vi "Request Data.vi"(6 "Qualifier":string, 8 "error in":errorcluster, 9 "notifier":refnum<notifier>, 10 "Data to Send":string, 11 "PRM in":refnum<class "PRM.lvclass">) -> (0 "error out":errorcluster, 3 "PRM out":refnum<class "PRM.lvclass">)   [LabVIEW 2019, in "PRM.lvlib" / "PRM.lvclass"]
doc: "Data to Send is a required input that describes the measurement or query function to be performed\nQualifier is a secondary variable used in the event that specificity must be provided to the query function\n****Note****\nIf further specificity is required, the qualifier must be used in a comma delimited format to increase the overall variable count. Additional specificity must be provided by the child class and interpreted by the automated call.\n\nnotifier is a single variant notifier in which the instrument will send the data notification to the automated tool."
uses:
  Library/PRM.lvclass
  C:/Users/Public/Documents/Development/builds/Instruments/Instruments.lvlibp/Library/Instruments.lvclass
  C:/Users/Public/Documents/Development/builds/Engine/Monitored Actor.lvlibp/Monitored Actor/Monitored Actor/Monitored Actor.lvclass
  builds/Instruments/Instruments.lvlibp/Private/Accessors/Read Poll(ms).vi
  builds/Instruments/Instruments.lvlibp/Accessors/Read Measured.vi
  <vilib>/Utility/error.llb/Error Cluster From Error Code.vi
  builds/Engine/Monitored Actor.lvlibp/Monitored Actor/Monitored Actor/Read Actor Label.vi
  builds/Instruments/Instruments.lvlibp/Private/Polymorphic/Special/Event from String.vi
  builds/Instruments/Instruments.lvlibp/Accessors/Command with Logging.vi
  <vilib>/ErrorRing/Error Ring.xnode
  builds/Instruments/Instruments.lvlibp/Library/Instruments.lvclass
  builds/Instruments/Instruments.lvlibp
  builds/Engine/Engine.lvlibp/Project/Engine.lvclass
  C:/Users/Public/Documents/Development/builds/Tools/Config.lvlibp/Config.lvclass
  C:/Users/Public/Documents/Development/builds/Engine/Engine.lvlibp/Project/Engine.lvclass
  C:/Users/Public/Documents/Development/builds/Engine/State Actor.lvlibp/Library/State Actor.lvclass
  C:/Users/Public/Documents/Development/builds/Engine/Panel Manager.lvlibp/Panel Actor/Panel Actor.lvclass
  C:/Users/Public/Documents/Development/builds/Engine/Actor Framework.lvlibp/1abvi3w/vi.lib/ActorFramework/Actor/Actor.lvclass
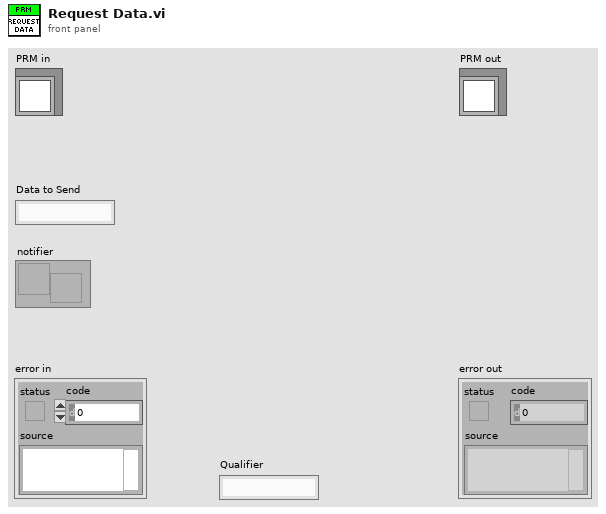
[diagram p1: front panel]
types:
  T1 = cluster{"Timestamp":timestamp, "Description":string, "Data":string}
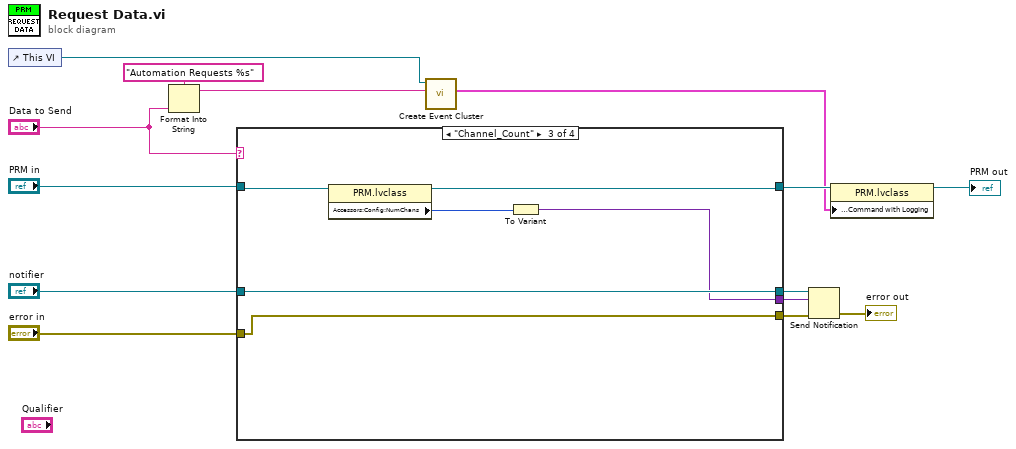
[diagram p0: block diagram]
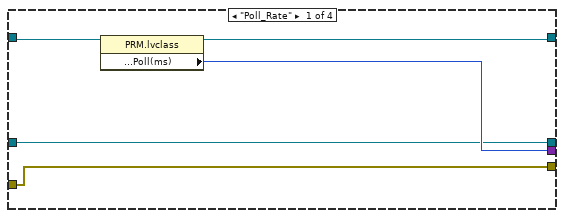
[diagram p2: hidden frame]
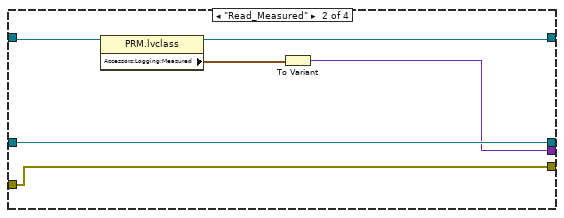
[diagram p3: hidden frame]
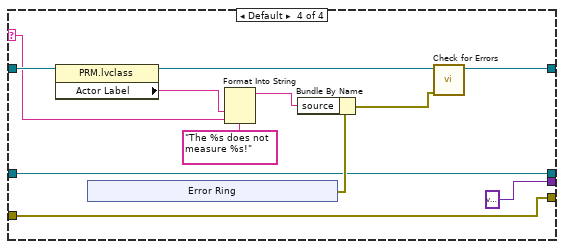
[diagram p4: hidden frame]
diagram:
  n1 = control-ref of="This VI"() -> (w14:refnum<vi>)
  n2 = Format Into String(format string="Automation Requests %s", "Data to Send") -> (resulting string=w12:string)  [unwired: 2 in, 1 out]
  n3 = case shown="\"Channel_Count\"" "Data to Send" {
    selector: "Data to Send" -> [_ _ _ w41]
    tunnel: "PRM in" -> [w19 w25 w31 w43]
    tunnel: [w17 w24 w30 w35] -> w10
    tunnel: [w18 w20 w26 variant] -> w6
    tunnel: "notifier" -> [w15 w22 w28 w33]
    tunnel: [w15 w22 w28 w33] -> w4
    tunnel: [w16 w23 w29 w32] -> w3
    tunnel: "error in" -> [w16 w23 w29 w32]
    frame "Poll_Rate" {
      n4 = property class="PRM.lvclass"(reference=w19) -> (reference out=w17:refnum<class "PRM.lvclass">, "Accessors:Configuration:Poll(ms)"=w18:u32)  [unwired: 1 in, 1 out]
    }
    frame "Read_Measured" {
      n5 = property class="PRM.lvclass"(reference=w25) -> (reference out=w24:refnum<class "PRM.lvclass">, "Accessors:Logging:Measured"=w21:waveform(dbl)[])  [unwired: 1 in, 1 out]
      n6 = To Variant(anything=w21) -> (Variant=w20:variant)
    }
    frame "Channel_Count" {
      n7 = property class="PRM.lvclass"(reference=w31) -> (reference out=w30:refnum<class "PRM.lvclass">, "Accessors:Config:NumChans"=w27:i32)  [unwired: 1 in, 1 out]
      n8 = To Variant(anything=w27) -> (Variant=w26:variant)
    }
    frame Default {
      n9 = property class="PRM.lvclass"(reference=w43) -> (reference out=w37:refnum<class "PRM.lvclass">, "Actor Label"=w42:string)  [unwired: 1 in, 1 out]
      n10 = xnode "Error Ring"() -> ("error out"=w39:errorcluster)
      n11 = Format Into String(format string="The %s does not measure %s!", w42, w41) -> (resulting string=w38:string)  [unwired: 2 in, 1 out]
      n12 = Bundle By Name(cluster=w39, "source"=w38) -> (w36:errorcluster)
      n13 = call "Check for Errors.vi"("error in"=w36, "Engine in"=w37) -> ("Engine out"=w35:refnum<class "PRM.lvclass">)  [unwired: 8 in, 1 out]
    }
  }
  n14 = call-poly "Create Event Cluster.vi"("Value"=w12, "VI Refnum"=w14) -> ("Event Data"=w8:T1)  [unwired: 9 in]
  n15 = Send Notification(notification=w6, notifier=w4, error in (no error)=w3) -> (error out=→"error out":errorcluster)  [unwired: 1 out]
  n16 = property class="PRM.lvclass"(reference=w10, "Accessors:Logging:Command with Logging"=w8) -> (reference out=→"PRM out":refnum<class "PRM.lvclass">)  [unwired: 1 in, 1 out]
